vi "VI Linearisierung v2.vi"() -> ()   [LabVIEW 2020, in "Linearisierung v2.lvlib"] (continued)
              n1351 = Bundle("PDF Optionen (Ausgang)"=w2317, "postprocess"=w2327, w2306, "Pfad Auto Lin"=w2304, "File Name LIN"=w2293, "Pfad LIN"=w2292, "LIN Filename override"=w2291) -> (w2337:T200)  [unwired: 1 in]
              n1352 = Increment(x=w2300) -> (x+1=w2347:i32)
              n1353 = call "Auto Filenames.vi"("Fehler (Eingang)"=w2356, "Flags Cluster"=w2337, "Zeitstempel"=w2338, "SpanInletClusterArray in"=w2333) -> ("Fehler (Ausgang)"=w2336:errorcluster, "LogInfo-Cluster"=w2351:T196, "Pfad LIN Cluster"=w2303:cluster{"Pfad LIN SPAN":T9, "Pfad LIN":path}, "SpanInletClusterArray out"=w2335:T19[], "Span_Name"=w2343:string, "File Names"=w2340:T197)  [unwired: 2 out]
              n1354 = call "get Polynom and EPA Auswahl from SPAN and Comp Index.vi"("Component Index"=w2300, "SPAN Idx"=w2301) -> ("Index Cluster"=w2297:T189, "EPA Optionsfeld out"=w2298:T2, "Polynom-Ordnung out"=w2299:T55)  [unwired: 7 in]
              n1355 = call "Set SPAN Component.vi"("Protocol_only"=TRUE, "Gasnummer"=w2347, "Autolin Hovacal (alt)"=w2330, "Daten Hovacal (alt)"=w2329) -> ("error out"=w2355:errorcluster, "Gaskomponente"=w2314:T7, "LogInfo-Einstellung-Cluster"=w2350:T190, "Komponente"=w2348:string, "Einheit in String"=w2339:string)  [unwired: 3 in]
              n1356 = Unbundle(w2303) -> ("Pfad LIN SPAN"=w2296:T9, "Pfad LIN"=w2302:path)
              n1357 = Bundle("Komponente"=w2348, w2347, "Einheit in String"=w2339) -> (w2316:T191)  [unwired: 1 in]
              n1358 = call "Set SPAN Component Tables.vi"("EPA Optionsfeld"=w2298, "Polynom-Ordnung"=w2299, "error in (no error)"=w2355, "Gaskomponente"=w2314, "postprocess"=w2327, "Tabellenref."=w2328) -> ("EPA Ausgangs-Cluster"=w2353:T193, "LIN Ausgangs-Cluster"=w2312:T194, "Daten Aufzeichnen Ausgangs-Cluster"=w2354:T195, "Aktiv EPA"=w2325:T57, "Aktiv LIN"=w2326:bool[])  [unwired: 1 out]
              n1359 = Unbundle By Name(w2340) -> ("LIN TXT Datei Name"=w2341:string)
              n1360 = call "get SPAN component params EPA LIN.vi"("Index in"=w2297, "LIN Ausgangs-Cluster"=w2312, "Gaskomponente"=w2314, "Component"=w2316) -> ("Component Cluster"=w2315:T199)  [unwired: 4 in, 3 out]
              n1361 = Unbundle By Name(w2354) -> ("Ausgabetabelle"=w2324:T53, "Eingabetabelle behandelt"=w2323:string[][])
              n1362 = Unbundle By Name(w2312) -> ("LIN Ausgabetabelle"=w2322:string[][], "XY-Graph"=w2321:cluster{dbl[], dbl[]}[], "Polynomkoeff."=w2313:T198)
              n1363 = Unbundle By Name(w2353) -> ("EPA Ausgabetabelle"=w2319:string[][], "XY-Graph"=w2320:cluster{dbl[], dbl[]}[], "LINVer Auswertung"=w2318:string[][])
              n1364 = call "Postprocess Wrapper next SPAN Comp.vi"("Fehler (Eingang, kein Fehler)"=w2336, "reprocessing"=w2327, "SpanInletClusterArray in"=w2335) -> ("Fehler (Ausgang)"=w2334:errorcluster, "active postprocessing SPAN Component"=w2332:i32, "active postprocessing SPAN"=w2331:i32, "SpanInletClusterArray out"=w2307:T19[], "last postprocessing SPAN"=w2294:bool)  [unwired: 4 in]
              n1365 = Not(x=w2308) -> (.not. x?=w2305:bool)
              n1366 = call "FGV SPAN Verriegelung.vi"("aktion"=Aktion_FGV_SPAN_Verriegelung."setcomp", "Component Cluster"=w2315) -> ()  [unwired: 7 in, 3 out]
              n1367 = call "get SPAN Table MG.vi"("automatisch in"=w2295, "active reprocessing SPAN"=w2301, "SpanInletClusterArray in"=w2307) -> ("SpanComponentInfos-Cluster"=w2310:T186)  [unwired: 2 in, 6 out]
              n1368 = case shown="True" w2346 {
                tunnel: w2296 -> [_ w2362]
                tunnel: w2351 -> [_ w2361]
                tunnel: w2350 -> [_ w2360]
                tunnel: w2345 -> [_ w2359]
                tunnel: w2344 -> [_ w2358]
                tunnel: [_ w2357] -> _
                frame False {
                }
                frame True {
                  # "Error Log"
                  n1369 = call "Log SPAN autorun Errors.vi"("Sprachliste"=w2358, "Component Infos"=w2359, "LogInfo-Einstellung-Cluster"=w2360, "LogInfo-Cluster"=w2361, "Pfad LIN"=w2362) -> ("error out"=w2357:errorcluster)  [unwired: 6 in]
                }
              }
              n1370 = Select(t=w2311, s=w2305, f=w2310) -> (s? t:f=w2309:T186)
            }
          }
          "XY-Graph LIN 2" <- w2193
          "XY-Graph EPA 2" <- w2191
          n1371 = Not(x=w2179) -> (.not. x?=w2173:bool)
          n1372 = local write "LIN Polynomkoeffizienten"(w2194) -> ()
          n1373 = And(x=w2173, y=w2174) -> (x .and. y?=w2175:bool)
          n1374 = local write "Pfad Auto Lin"(w2159) -> ()
          n1375 = local write "Aktiv LIN"(w2199) -> ()
          n1376 = local write "Aktiv"(w2198) -> ()
          n1377 = local write "Ausgabetabelle"(w2197) -> ()
          n1378 = local write "Eingabetabelle"(w2196) -> ()
          n1379 = local write "LIN Ausgabetabelle"(w2195) -> ()
          n1380 = local write "XY-Graph LIN"(w2193) -> ()
          n1381 = local write "EPA Ausgabetabelle"(w2192) -> ()
          n1382 = local write "XY-Graph EPA"(w2191) -> ()
          n1383 = local write "EPA Auswertung"(w2190) -> ()
          n1384 = control-ref of="XY-Graph LIN 2"() -> (w2216:refnum<vi>)
          n1385 = control-ref of="XY-Graph EPA 2"() -> (w2215:refnum<vi>)
          n1386 = Select(t=w2176, s=w2175, f=w2178) -> (s? t:f=w2177:bool)
          n1387 = And(x=w2204, y=w2176) -> (x .and. y?=w2205:bool)
          n1388 = Bundle("SpanComponentInfos-Cluster"=w2181, "Span_Name"=w2211) -> (w2210:T201)  [unwired: 1 in]
          n1389 = case shown="False" w2205 {
            tunnel: w2209 -> [_ w2229]
            tunnel: [_ w2227] -> w2207
            tunnel: w2164 -> [w2221 w2228]
            tunnel: [w2221 w2226] -> w2158
            tunnel: w2206 -> [_ w2222]
            frame False {
            }
            frame True {
              n1390 = call "LIN speichern.vi"("File Name LIN"=w2229, "Pfad LIN"=w2228) -> ("error out"=w2227:errorcluster, ".LIN Datei Pfad"=w2224:path, "Pfad LIN out"=w2226:T9)  [unwired: 7 in]
              n1391 = Bundle("active postprocessing SPAN"=w2222, ".LIN Datei Pfad"=w2224) -> (w2223:T202)  [unwired: 1 in]
              n1392 = call "FGV Post Processing.vi"("Aktion"=Aktion_FGV_Post_Processing."filenames", "filenemas Cluster"=w2223) -> ()  [unwired: 6 in, 4 out]
            }
          }
          n1393 = Bundle("XY-Graph LIN 2"=w2216, "XY-Graph EPA 2"=w2215, "ResultPictures"=w2171, w2161) -> (w2214:T203)  [unwired: 1 in]
          n1394 = And(x=w2176, y=w2177) -> (x .and. y?=w2189:bool)
          n1395 = Select(t=enum16{"LIN", "EPA", "LIN + EPA"}."LIN", s=w2155, f=enum16{"LIN", "EPA", "LIN + EPA"}."LIN + EPA" ("LIN/EPA")) -> (s? t:f=w2156:enum16{"LIN", "EPA", "LIN + EPA"})
          n1396 = Select(t=w2156, s=w2163, f=enum16{"LIN", "EPA", "LIN + EPA"}."LIN" ("LIN/EPA")) -> (s? t:f=w2170:enum16{"LIN", "EPA", "LIN + EPA"})
          n1397 = Select(t=enum16{"LIN", "EPA", "LIN + EPA"}."EPA", s=w2160, f=w2170) -> (s? t:f=w2168:enum16{"LIN", "EPA", "LIN + EPA"})
          n1398 = call "PDF Protokolle gemeinsam.vi"("start"=w2189, "LIN/EPA"=w2168, "Pfad LIN"=w2158, "File Names"=w2208, "Graphs"=w2214, "Fehler (Eingang, kein Fehler)"=w2207, "SpanComponentInfos-Cluster"=w2210, "PDF Optionen"=w2183, "Polynom-Ordnung"=w2188) -> ("Fehler (Ausgang)"=w2166:errorcluster, "EPA Context (Ausgang)"=w2212:refnum<class "Context.lvclass">, "Context (Ausgang)"=w2213:refnum<class "Context.lvclass">)
          n1399 = call "FGV SPAN Verriegelung.vi"("aktion"=Aktion_FGV_SPAN_Verriegelung."Reset Save EPA redirect", "error in (no error)"=w2166) -> ("error out"=w2165:errorcluster)  [unwired: 7 in, 2 out]
        }
        n1400 = Not(x=w2038) -> (.not. x?=w2036:bool)
        n1401 = Not(x=w2037) -> (.not. x?=w2035:bool)
        n1402 = And(x=w2036, y=w2035) -> (x .and. y?=w2034:bool)
        n1403 = case shown="True" w2068 {
          tunnel: w2079 -> [w2379 _]
          tunnel: w2057 -> [_ w2399]
          tunnel: w2078 -> [w2374 w2397]
          tunnel: w2076 -> [w2364 w2396]
          tunnel: w2075 -> [w2363 w2395]
          tunnel: w2074 -> [w2377 w2394]
          tunnel: w2039 -> [_ w2393]
          tunnel: [w2373 _] -> _
          tunnel: w2060 -> [w2372 w2392]
          tunnel: w2067 -> [w2369 _]
          tunnel: w2066 -> [_ w2391]
          tunnel: w2066 -> [_ w2390]
          tunnel: w2048 -> [_ w2389]
          tunnel: w2038 -> [w2367 _]
          tunnel: w2044 -> [w2368 _]
          tunnel: w2043 -> [_ w2388]
          tunnel: w2034 -> [_ w2387]
          frame False {
            # "manuell"
            n1404 = Not(x=w2367) -> (.not. x?=w2365:bool)
            n1405 = case shown="Kein Fehler" w2369 {
              tunnel: ["Daten gespeichert!" ("String") "Fehler beim schreiben der Daten" ("String")] -> w2378
              frame No Error {
              }
              frame Error {
              }
            }
            n1406 = call "FGV SPAN Verriegelung.vi"("aktion"=Aktion_FGV_SPAN_Verriegelung."unlock") -> ("error out"=w2370:errorcluster)  [unwired: 8 in, 2 out]
            n1407 = Select(t=w2364, s=w2365, f=w2363) -> (s? t:f=w2366:refnum<class "Context.lvclass">)
            n1408 = call "ClosePage.vi"("popup viewer"=w2372, "Fehler (Eingang, kein Fehler)"=w2377, "Context (Eingang)"=w2366) -> ("Fehler (Ausgang)"=w2373:errorcluster)  [unwired: 8 in]
            n1409 = property class="Bool."(reference=w2374, error in=w2370, "DisabledEnum"=T66."Disabled and Grayed Out" ("Deaktiviert")) -> (error out=w2376:errorcluster)  [unwired: 1 out]
            n1410 = disable-structure shown="Deaktiviert" {
              disable-tunnel: w2368 -> [w2382 _]
              disable-tunnel: w2367 -> [w2381 _]
              frame Disabled {
                n1411 = case shown="False" w2381 {
                  tunnel: w2382 -> [w2383 w2384]
                  frame False {
                    n1412 = local write "Pfad LIN"(w2383) -> ()
                  }
                  frame True {
                    n1413 = local write "EPA Pfad"(w2384) -> ()
                  }
                }
              }
              frame Enabled {
              }
            }
            n1414 = call <vilib>:"Clear Errors.vi"("error in (no error)"=w2376) -> ()  [unwired: 5 in, 2 out]
            n1415 = call "Texte in VIs uebersetzen.vi"("Sprachliste"=w2379, "String zum Übersetzen"=w2378) -> ("String zum Übersetzen"=w2380:string)  [unwired: 9 in, 4 out]
            n1416 = One Button Dialog(message=w2380) -> ()  [unwired: 1 in, 1 out]
          }
          frame True {
            # "automatisch"
            n1417 = case shown="False" w2391 {
              tunnel: [Aktion_FGV_Spans_abarbeiten."lesen" ("Aktion") Aktion_FGV_Spans_abarbeiten."next" ("Aktion")] -> w2402
              frame False {
              }
              frame True {
              }
            }
            n1418 = call "FGV Spans abarbeiten.vi"("Aktion"=w2402, "SpanInletClusterArray in"=w2399) -> ("Comp Idx out"=w2398:i32, "active SPAN Idx out"=w2400:i32)  [unwired: 4 in, 4 out]
            n1419 = Less Than 0?(x=w2400) -> (x < 0?=w2401:bool)
            n1420 = case shown="True" w2401 {
              tunnel: w2398 -> [_ _]
              tunnel: w2397 -> [_ w2435]
              tunnel: w2396 -> [w2411 w2429]
              tunnel: w2395 -> [w2410 w2428]
              tunnel: w2394 -> [w2409 w2430]
              tunnel: w2393 -> [w2408 w2424]
              tunnel: [w2406 w2426] -> _
              tunnel: [w2407 w2427] -> _
              tunnel: [_ w2434] -> _
              tunnel: w2392 -> [w2405 w2431]
              tunnel: w2390 -> [_ w2432]
              tunnel: w2389 -> [_ w2423]
              tunnel: w2388 -> [_ w2422]
              tunnel: w2387 -> [_ w2421]
              frame False {
                # "weiter"
                n1421 = case shown="True" w2408 {
                  tunnel: w2411 -> [_ w2420]
                  tunnel: w2410 -> [_ w2419]
                  tunnel: w2409 -> [w2414 w2418]
                  tunnel: [w2414 w2417] -> w2407
                  tunnel: [w2414 w2416] -> w2406
                  tunnel: w2405 -> [_ w2415]
                  frame False {
                  }
                  frame True {
                    n1422 = call "ClosePage.vi"("popup viewer"=w2415, "Fehler (Eingang, kein Fehler)"=w2418, "Context (Eingang)"=w2420) -> ("Fehler (Ausgang)"=w2417:errorcluster)  [unwired: 8 in]
                    n1423 = call "ClosePage.vi"("popup viewer"=w2415, "Fehler (Eingang, kein Fehler)"=w2418, "Context (Eingang)"=w2419) -> ("Fehler (Ausgang)"=w2416:errorcluster)  [unwired: 8 in]
                  }
                }
                n1424 = property on="STARTEN" class="Bool. (strikt)"("Val(Sgnl)"=T4 TRUE ("Wert (signalisierend)")) -> (error out=w2412:errorcluster)  [unwired: 2 in, 1 out]
                n1425 = call <vilib>:"Clear Errors.vi"("error in (no error)"=w2412) -> ()  [unwired: 5 in, 2 out]
              }
              frame True {
                # "fertig"
                n1426 = call "FGV Spans abarbeiten.vi"("Aktion"=Aktion_FGV_Spans_abarbeiten."idle") -> ("error out"=w2433:errorcluster)  [unwired: 5 in, 5 out]
                n1427 = Or(x=w2423, y=w2424) -> (x .or. y?=w2425:bool)
                n1428 = case shown="False" w2432 {
                  tunnel: [w2447 w2471] -> w2434
                  tunnel: w2433 -> [w2448 w2470]
                  tunnel: w2431 -> [w2445 w2468]
                  tunnel: w2430 -> [w2444 w2465]
                  tunnel: w2429 -> [w2446 w2467]
                  tunnel: w2428 -> [w2443 w2466]
                  tunnel: [w2442 w2464] -> w2427
                  tunnel: [w2441 w2463] -> w2426
                  tunnel: w2425 -> [w2440 _]
                  tunnel: w2422 -> [_ w2462]
                  tunnel: w2421 -> [w2439 _]
                  frame False {
                    # "reprocessing next \noder fertig"
                    n1429 = case shown="False" w2439 {
                      tunnel: w2448 -> [w2450 w2453]
                      tunnel: [w2449 w2452] -> w2447
                      frame True {
                        n1430 = call "FGV Post Processing.vi"("Aktion"=Aktion_FGV_Post_Processing."next", "error in (no error)"=w2450) -> ("error out"=w2449:errorcluster)  [unwired: 6 in, 3 out]
                      }
                      frame False {
                        n1431 = call "FGV Post Processing.vi"("Aktion"=Aktion_FGV_Post_Processing."same", "error in (no error)"=w2453) -> ("error out"=w2452:errorcluster)  [unwired: 6 in, 3 out]
                      }
                    }
                    n1432 = case shown="True" w2440 {
                      tunnel: w2446 -> [_ w2461]
                      tunnel: w2445 -> [_ w2460]
                      tunnel: w2444 -> [w2455 w2459]
                      tunnel: w2443 -> [_ w2458]
                      tunnel: [w2455 w2457] -> w2442
                      tunnel: [w2455 w2456] -> w2441
                      frame False {
                      }
                      frame True {
                        n1433 = call "ClosePage.vi"("popup viewer"=w2460, "Fehler (Eingang, kein Fehler)"=w2459, "Context (Eingang)"=w2461) -> ("Fehler (Ausgang)"=w2457:errorcluster)  [unwired: 8 in]
                        n1434 = call "ClosePage.vi"("popup viewer"=w2460, "Fehler (Eingang, kein Fehler)"=w2459, "Context (Eingang)"=w2458) -> ("Fehler (Ausgang)"=w2456:errorcluster)  [unwired: 8 in]
                      }
                    }
                  }
                  frame True {
                    # "start\nreprocessing"
                    n1435 = local write "Pfad LIN"(w2462) -> ()
                    n1436 = local write "EPA Pfad"(w2462) -> ()
                    n1437 = call "FGV Post Processing.vi"("Aktion"=Aktion_FGV_Post_Processing."enable", "error in (no error)"=w2470) -> ("error out"=w2471:errorcluster)  [unwired: 6 in, 3 out]
                    n1438 = call "ClosePage.vi"("popup viewer"=w2468, "Fehler (Eingang, kein Fehler)"=w2465, "Context (Eingang)"=w2467) -> ("Fehler (Ausgang)"=w2464:errorcluster)  [unwired: 8 in]
                    n1439 = call "ClosePage.vi"("popup viewer"=w2468, "Fehler (Eingang, kein Fehler)"=w2465, "Context (Eingang)"=w2466) -> ("Fehler (Ausgang)"=w2463:errorcluster)  [unwired: 8 in]
                  }
                }
                n1440 = property class="Bool."(reference=w2435, "DisabledEnum"=T66."Disabled and Grayed Out" ("Deaktiviert")) -> (error out=w2437:errorcluster)  [unwired: 1 in, 1 out]
                n1441 = call <vilib>:"Clear Errors.vi"("error in (no error)"=w2437) -> ()  [unwired: 5 in, 2 out]
              }
            }
          }
        }
      }
      event Value Change {
        n1442 = event-data() -> ()  [unwired: 1 in, 1 out]
        n1443 = local read "Aktiv"() -> (w2482:T57)
        n1444 = call "EPA aktiv genug Punkte.vi"("Aktiv"=w2482) -> ()  [unwired: 9 in, 2 out]
        n1445 = case shown="True" TRUE {
          tunnel: w2478 -> [_ w2494]
          tunnel: w2477 -> [_ w2493]
          tunnel: w2476 -> [_ w2492]
          tunnel: w2475 -> [_ w2491]
          tunnel: w2474 -> [_ w2488]
          tunnel: w2473 -> [w2483 _]
          frame False {
            n1446 = call "Texte in VIs uebersetzen.vi"("Sprachliste"=w2483, "String zum Übersetzen"="EPA Test nicht gültig!\nMindestens 10 aktive Punkte nötig.\nPDF wurde nicht erzeugt" ("Nachricht")) -> ("String zum Übersetzen"=w2484:string)  [unwired: 9 in, 4 out]
            n1447 = One Button Dialog(message=w2484) -> ()  [unwired: 1 in, 1 out]
          }
          frame True {
            # "immer, auch wenn weniger als 10, wird im PDF eh angezeigt !"
            n1448 = call "Postprocessing aktiv.vi"() -> ("postprocess"=w2486:bool)  [unwired: 10 in, 1 out]
            n1449 = case shown="True" TRUE {
              tunnel: w2494 -> [_ _]
              tunnel: w2493 -> [_ _]
              tunnel: w2492 -> [_ _]
              tunnel: w2491 -> [_ _]
              tunnel: "EPA Pfad" -> [_ _]
              tunnel: "EPA Filename" -> [_ _]
              tunnel: w2488 -> [_ _]
              tunnel: w2486 -> [_ _]
              frame False {
                # "manuell - jetzt auch automatisiert !"
              }
              frame True {
                # "postprocessing ... wird im automatic abgehandelt (LIN Speichern)\n#EPA_Save_redirect\nNur mehr hier, da Postprocessing jetzt alles auf einmal speichert - EPA Speichern dann deaktiviert !\nUnd manuell geht auch mit Pfad in auto speichern ... der Dateiname wird soweiso nie genommen (aber dann angezeigt).\nmit #LinV2_auto_singleSave hier wieder aktiv ..."
                n1450 = call "FGV SPAN Verriegelung.vi"("aktion"=Aktion_FGV_SPAN_Verriegelung."Set Save EPA redirect") -> ("error out"=w2495:errorcluster)  [unwired: 8 in, 2 out]
                n1451 = property on="Speichern LIN" class="Bool. (strikt)"(error in=w2495, "Val(Sgnl)"=T4 TRUE ("Wert (signalisierend)")) -> (error out=w2498:errorcluster)  [unwired: 1 in, 1 out]
                n1452 = call <vilib>:"Clear Errors.vi"("error in (no error)"=w2498) -> ()  [unwired: 5 in, 2 out]
              }
            }
          }
        }
      }
      event Value Change {
        # "#LinV2_auto_singleSave"
        n1453 = event-data() -> ()  [unwired: 1 in, 6 out]
        n1454 = local read "Gasnummer LIN"() -> (w2501:T49)
        n1455 = Decrement(x=w2501) -> (x-1=w2502:T49)
        n1456 = call "MG FileName.vi"("Gasnummer:"=w2502) -> ("LIN TXT Datei Name"=w2503:string, "EPA TXT Datei Name"=w2504:string)  [unwired: 7 in, 2 out]
        n1457 = call "Preset Filenames.vi"("FileNameInput References"=w2499, "Filename Flag Cluster"=w2500, "LIN TXT Datei Name"=w2503, "EPA TXT Datei Name"=w2504) -> ()  [unwired: 8 in]
      }
      event Value Change {
        w2508 = T1 TRUE ("Wert")
        # "#LinV2_auto_singleSave"
        n1458 = event-data() -> ()  [unwired: 1 in, 6 out]
        n1459 = Unbundle(w2513) -> ("LIN Filename override"=w2512:refnum<vi>, "EPA Filename override"=w2511:refnum<vi>)
        n1460 = property class="Bool. (strikt)"(reference=w2512, "Value"=w2508) -> (error out=w2510:errorcluster)  [unwired: 1 in, 1 out]
        n1461 = property class="Bool. (strikt)"(reference=w2511, error in=w2510, "Value"=w2508) -> (error out=w2509:errorcluster)  [unwired: 1 out]
        n1462 = call <vilib>:"Clear Errors.vi"("error in (no error)"=w2509) -> ()  [unwired: 5 in, 2 out]
      }
      event Value Change {
        # "#Option10xSpanAuto ???"
        n1463 = event-data() -> ()  [unwired: 1 in, 1 out]
        n1464 = call "LinDaten speichern und laden.vi"("Aktion"=enum16{"speichern", "laden"}."speichern") -> ("error out"=w2527:errorcluster, "Setup Daten-Cluster"=w2520:T204)  [unwired: 4 in, 5 out]
        n1465 = Unbundle By Name(w2520) -> ("[Analyser]"=w2519:string)
        n1466 = call "LinDaten speichern und laden.vi"("Aktion"=enum16{"speichern", "laden"}."laden", "error in (no error)"=w2527, "test Polynom"=TRUE, "Analysator"=w2519) -> ("error out"=w2530:errorcluster, "LIN Protokoll Daten"=w2533:T119, "MessDaten Array"=w2532:string[][][], "Ident Cluster"=w2531:T205, "Setup Daten-Cluster"=w2525:T204, "Settings Cluster"=w2517:T206)  [unwired: 1 in, 1 out]
        n1467 = call "LIN Laden Errors.vi"("Fehler (Eingang, kein Fehler)"=w2530, "Ident Cluster"=w2531) -> ("error out"=w2529:errorcluster, "Error orccured"=w2526:bool, "LIN Loading Error Description Array"=w2524:T207, "Ident Cluster out"=w2523:T205)  [unwired: 5 in, 1 out]
        n1468 = case shown="True" w2526 {
          tunnel: w2520 -> [_ w2575]
          tunnel: w2525 -> [_ w2576]
          tunnel: w2524 -> [_ _]
          tunnel: w2523 -> [_ w2574]
          tunnel: [w2572 w2573] -> w2522
          frame False {
            w2572 = T4 TRUE  # CONTINUE
          }
          frame True {
            n1469 = call "show LIN Load Errors.vi"("loaded Setup Daten-Cluster"=w2576, "Ident Cluster"=w2574, "local Setup Daten-Cluster"=w2575) -> ("CONTINUE"=w2573:T4)  [unwired: 8 in]
          }
        }
        n1470 = case shown="True" w2522 {
          tunnel: w2533 -> [_ w2549]
          tunnel: w2532 -> [_ w2547]
          tunnel: w2529 -> [_ w2545]
          tunnel: w2517 -> [_ w2537]
          frame False {
          }
          frame True {
            # "Wie hier mit anderem Polynom verfahren ... und für MG alle Komp !?\nHier auswerten und Fehlermeldung ?!\nOder auch reinrechnen ?\n#Lin_Load_Polynom_Question"
            n1471 = call "Lin Daten aufarbeiten.vi"("Lin-Polynom"=w2549, "error in (no error)"=w2545, "Aktionen"=Aktion_Lin_Daten_aufarbeiten."Protkolldaten") -> ("error out"=w2548:errorcluster)  [unwired: 14 in, 10 out]
            n1472 = call "Lin Daten aufarbeiten.vi"("error in (no error)"=w2548, "TabellenArray"=w2547, "Aktionen"=Aktion_Lin_Daten_aufarbeiten."Nachbehandlung laden") -> ("error out"=w2546:errorcluster)  [unwired: 14 in, 10 out]
            n1473 = call "Komponentenausgabe.vi"("error in (no error)"=w2546) -> ("error out"=w2555:errorcluster, "Gaskomponente"=w2554:T7)  [unwired: 7 in, 2 out]
            n1474 = call "Lin Daten aufarbeiten.vi"("Index (Seite)"=w2554, "error in (no error)"=w2555, "Aktionen"=Aktion_Lin_Daten_aufarbeiten."lesen") -> ("TabellenArray"=w2553:string[][][], "Lin-Polynom"=w2538:T119, "error out"=w2539:errorcluster)  [unwired: 14 in, 8 out]
            n1475 = disable-structure shown="Deaktiviert" {
              disable-tunnel: w2553 -> [w2562 _]
              disable-tunnel: [w2558 w2568] -> w2543
              disable-tunnel: w2539 -> [w2557 w2569]
              disable-tunnel: w2538 -> [_ w2571]
              disable-tunnel: w2537 -> [_ w2570]
              frame Disabled {
                n1476 = for {
                  tunnel: w2562 -> [w2567] mode=indexing
                  tunnel: [w2563] -> w2560
                  stop <- w2564 stop-if-true
                  n1477 = call "Tabelle initialisieren.vi"("Neue Tabelle"=w2567) -> ("Tabelle"=w2566:string[][])  [unwired: 10 in]
                  n1478 = Array Size(array=w2566) -> (size(s)=w2565:i32[])
                  n1479 = Index Array(array=w2565) -> (element=w2563:i32)  [unwired: 1 in]
                  n1480 = Not Equal To 0?(x=w2563) -> (x != 0?=w2564:bool)
                }
                n1481 = call "LIN_EPA aktiv setzen.vi"("Anzahl aktiv"=w2560) -> ("Aktiv"=w2559:bool[][])  [unwired: 9 in, 1 out]
                n1482 = call "Lin Daten aufarbeiten.vi"("error in (no error)"=w2557, "LINArray"=w2559, "Aktionen"=Aktion_Lin_Daten_aufarbeiten."LIN/EPA aktiv laden", "EPA Array"=w2559) -> ("error out"=w2558:errorcluster)  [unwired: 13 in, 10 out]
              }
              frame Enabled {
                n1483 = call "LIN Laden nur Aktiv setzen.vi"("error in (no error)"=w2569, "LIN Protokoll Daten"=w2571, "Settings Cluster new"=w2570) -> ("error out"=w2568:errorcluster)  [unwired: 8 in]
              }
            }
            n1484 = control-ref of="passive Komponente:"() -> (w2544:refnum<vi>)
            n1485 = property class="Ring (strikt)"(reference=w2544, error in=w2543, "DisabledEnum"=T66."Enabled" ("Deaktiviert")) -> (error out=w2542:errorcluster)  [unwired: 1 out]
            n1486 = property on="Gasnummer Generieren" class="DigWert (strikt)"(error in=w2542, "Val(Sgnl)"=T49 1 ("Wert (signalisierend)")) -> (error out=w2540:errorcluster)  [unwired: 1 in, 1 out]
            n1487 = call <vilib>:"Clear Errors.vi"("error in (no error)"=w2540) -> ()  [unwired: 5 in, 2 out]
          }
        }
      }
      event Value Change {
        # "#LIN_only_save_Polynoms"
        n1488 = event-data() -> ()  [unwired: 1 in, 1 out]
        n1489 = call "Komponentenausgabe.vi"() -> ("Gaskomponente"=w2589:T7)  [unwired: 8 in, 3 out]
        n1490 = call "Lin Daten aufarbeiten.vi"("Index (Seite)"=w2589, "Aktiv"="Aktiv", "Aktionen"=Aktion_Lin_Daten_aufarbeiten."EPA aktiviert") -> ("Index (Seite) out"=w2582:i32, "error out"=w2590:errorcluster)  [unwired: 14 in, 9 out]
        n1491 = call "aktueller SPAN und Komponent Index.vi"() -> ("akt SPAN out"=w2577:i32)  [unwired: 7 in, 4 out]
        n1492 = call "LIN Polynom Ordnung oder Aktiv Changes für Postprocessing.vi"("Aktion"=Aktion_LIN_Polynom_Ordnung_ode_Aktiv_Changes_für_Postprocessing."schreiben", "active SPAN Idx"=w2577, "Changes"=TRUE) -> ()  [unwired: 5 in, 4 out]
        n1493 = call "Lin Daten aufarbeiten.vi"("Index (Seite)"=w2582, "error in (no error)"=w2590, "Aktionen"=Aktion_Lin_Daten_aufarbeiten."EPA auswerten") -> ("Index (Seite) out"=w2581:i32, "error out"=w2598:errorcluster)  [unwired: 14 in, 9 out]
        n1494 = call "Lin Daten aufarbeiten.vi"("Index (Seite)"=w2581, "error in (no error)"=w2598, "Aktionen"=Aktion_Lin_Daten_aufarbeiten."lesen") -> ("Eingabetabelle"=w2596:T54, "EPA Auswertung"=w2584:cluster{sgl[], sgl[], bool[]}, "error out"=w2597:errorcluster)  [unwired: 14 in, 8 out]
        n1495 = call "EPA_Tabelle zusammenbauen.vi"("error in (no error)"=w2597, "Eingabetabelle"=w2596) -> ("error out"=w2592:errorcluster, "XY-Graph"=w2593:cluster{dbl[], dbl[]}[], "EPA Ausgabetabelle"=w2595:string[][])  [unwired: 7 in]
        n1496 = control-ref of="EPA Auswertung"() -> (w2586:refnum<vi>)
        n1497 = call "FGV Auswertung sammeln.vi"("Aktion"=Aktion_FGV_Auswertung_sammeln."lesen", "error in (no error)"=w2592) -> ("LINVer Auswertung"=w2591:string[][])  [unwired: 7 in, 2 out]
        n1498 = Unbundle(w2584) -> (w2585:bool[])  [unwired: 2 out]
        n1499 = local write "EPA Ausgabetabelle"(w2595) -> ()
        n1500 = local write "EPA Auswertung"(w2591) -> ()
        n1501 = local write "XY-Graph EPA"(w2593) -> ()
        n1502 = call "Zellen einfaerben.vi"("Färben"=w2585, "Tabellenref."=w2586) -> ()  [unwired: 10 in]
      }
      event Value Change {
        # "#LIN_only_save_Polynoms"
        n1503 = event-data() -> ()  [unwired: 1 in, 1 out]
        n1504 = local read "Polynom-Ordnung"() -> (w2619:T55)
        n1505 = call "Komponentenausgabe.vi"() -> ("Gaskomponente"=w2614:T7)  [unwired: 8 in, 3 out]
        n1506 = call "aktueller SPAN und Komponent Index.vi"() -> ("akt SPAN out"=w2602:i32)  [unwired: 7 in, 4 out]
        n1507 = call "Lin Daten aufarbeiten.vi"("Index (Seite)"=w2614, "Aktiv"="Aktiv LIN", "Aktionen"=Aktion_Lin_Daten_aufarbeiten."LIN aktiviert") -> ("Index (Seite) out"=w2607:i32, "error out"=w2618:errorcluster)  [unwired: 14 in, 9 out]
        n1508 = call "LIN Polynom Ordnung oder Aktiv Changes für Postprocessing.vi"("Aktion"=Aktion_LIN_Polynom_Ordnung_ode_Aktiv_Changes_für_Postprocessing."schreiben", "active SPAN Idx"=w2602, "Changes"=TRUE) -> ()  [unwired: 5 in, 4 out]
        n1509 = call "Lin Daten aufarbeiten.vi"("Index (Seite)"=w2607, "error in (no error)"=w2618, "Polynom-Ordnung"=w2619, "Aktionen"=Aktion_Lin_Daten_aufarbeiten."Lin auswerten") -> ("Index (Seite) out"=w2606:i32, "error out"=w2617:errorcluster)  [unwired: 13 in, 9 out]
        n1510 = call "Lin Daten aufarbeiten.vi"("Index (Seite)"=w2606, "error in (no error)"=w2617, "Aktionen"=Aktion_Lin_Daten_aufarbeiten."lesen") -> ("Eingabetabelle"=w2615:T54, "Lin-Polynom"=w2612:T119)  [unwired: 14 in, 9 out]
        n1511 = Unbundle By Name(w2612) -> ("Polynomkoeff."=w2610:dbl[])
        n1512 = call "LinTabelle zusammenbauen.vi"("Eingabetabelle"=w2615) -> ("LIN Ausgabetabelle"=w2621:string[][])  [unwired: 7 in, 3 out]
        n1513 = Array To Cluster(array=w2610) -> (cluster=w2611:T185)
        n1514 = local write "LIN Polynomkoeffizienten"(w2611) -> ()
        n1515 = local write "LIN Ausgabetabelle"(w2621) -> ()
      }
      event "Boolsch für LinStart": Value Change {
        # "#Option10xSpanAuto"
        n1516 = event-data() -> ()  [unwired: 1 in, 1 out]
        n1517 = call "Test Status.vi"("Aktion"=Aktion_Test_Status."lesen") -> ("Tests sperren"=w2624:bool)  [unwired: 11 in, 3 out]
        n1518 = local read "Anforderung"() -> (w2626:T4)
        n1519 = control-ref of="Anforderung"() -> (w2631:refnum<vi>)
        n1520 = control-ref of="Status"() -> (w2630:refnum<vi>)
        n1521 = Not(x=w2624) -> (.not. x?=w2623:bool)
        n1522 = Or(x="Boolsch für LinStart", y="STARTEN") -> (x .or. y?=w2647:T4)
        n1523 = Compound Arithmetic op=AND ("Mehrfacharithmetik")(w2647, w2626, w2623) -> (w2641:T4)
        n1524 = property class="Bool."(reference=w2645, "DisabledEnum"=T66."Enabled" ("Deaktiviert")) -> (error out=w2644:errorcluster)  [unwired: 1 in, 1 out]
        n1525 = Bundle By Name(cluster=T152 {"Stufen Tabelle Array"=[], "auto Scan Points"=[], "Punkte umkehren"=[], "Parameterkontrolle Array"=[], "Eingabetabelle"=refnum, "Ausgabetabelle"=refnum, "Anforderung"=refnum, "Status Str Referenz"=refnum, "Prüfgasnamen Array"=[]} ("Referenzen Cluster"), "Stufen Tabelle Array"=w2638, "auto Scan Points"=w2637, "Punkte umkehren"=w2636, "Parameterkontrolle Array"=w2635, "Eingabetabelle"=w2634, "Ausgabetabelle"=w2632, "Anforderung"=w2631, "Status Str Referenz"=w2630, "Prüfgasnamen Array"=w2627) -> (w2633:T152)
        n1526 = case shown="False" w2642 {
          tunnel: [w2654 TRUE] -> w2646
          tunnel: w2641 -> [w2654 _]
          frame False {
          }
          frame True {
            # "#TestRun"
          }
        }
        n1527 = call "FGV Stoerungen sammeln und auswerten.vi"("Aktion"=Aktion_FGV_Stoerungen_sammeln_und_auswerten."lesen") -> ("Error"=w2650:bool)  [unwired: 12 in, 6 out]
        n1528 = call <vilib>:"Clear Errors.vi"("error in (no error)"=w2644) -> ()  [unwired: 5 in, 2 out]
        n1529 = case shown="True" w2646 {
          selector: w2646 -> [_ w2676]
          tunnel: w2652 -> [w2659 w2674]
          tunnel: w2650 -> [_ w2677]
          tunnel: w2636 -> [_ w2675]
          tunnel: [T4 FALSE ("STARTEN") _] -> w2640
          tunnel: w2633 -> [_ w2673]
          tunnel: w2630 -> [_ w2672]
          tunnel: w2626 -> [w2657 _]
          frame False {
            n1530 = case shown="True" w2657 {
              tunnel: w2659 -> [w2665 w2671]
              tunnel: [w2660 w2666] -> w2656
              frame False {
                # "keine Anforderung GD"
                n1531 = call "Texte in VIs uebersetzen.vi"("Sprachliste"=w2665, "String zum Übersetzen"="Keine Anforderung Gasteiler!" ("Status")) -> ("String zum Übersetzen"=w2661:string)  [unwired: 9 in, 4 out]
                n1532 = call "FGV Daten Abholung uebergeben.vi"("Zustand"=w2661, "Beendet"=FALSE, "Aktion"=Aktion_FGV_Daten_Abholung_uebergebenctl."schreiben") -> ("Zustand"=w2660:string)  [unwired: 8 in, 4 out]
              }
              frame True {
                # "anderer Test läuft gerade"
                n1533 = call "Texte in VIs uebersetzen.vi"("Sprachliste"=w2671, "String zum Übersetzen"="Anderer Test läuft gerade.\nBitte etwas Geduld." ("Status")) -> ("String zum Übersetzen"=w2667:string)  [unwired: 9 in, 4 out]
                n1534 = call "FGV Daten Abholung uebergeben.vi"("Zustand"=w2667, "Beendet"=FALSE, "Aktion"=Aktion_FGV_Daten_Abholung_uebergebenctl."schreiben") -> ("Zustand"=w2666:string)  [unwired: 8 in, 4 out]
              }
            }
            n1535 = local write "Status"(w2656) -> ()
          }
          frame True {
            n1536 = stacked-sequence {
              seq-local: [_ w2699 _ _ _ _] -> [_ _ w2792 w2818 w2827 _]
              tunnel: w2677 -> [w2682 _ _ _ _ _]
              tunnel: w2676 -> [w2681 _ _ _ _ _]
              tunnel: w2675 -> [_ w2710 _ _ _ _]
              tunnel: w2674 -> [_ w2700 _ _ _ _]
              tunnel: w2673 -> [_ w2697 _ _ _ _]
              tunnel: w2672 -> [_ w2706 _ _ _ _]
              frame #0 {
                w2683 = ""
                # "#Option10xSpanAuto"
                n1537 = disable-structure shown="Aktiviert" {
                  disable-tunnel: w2682 -> [w2687 _]
                  disable-tunnel: w2681 -> [w2686 _]
                  frame Disabled {
                    n1538 = And(x=w2687, y=w2686) -> (x .and. y?=w2691:bool)
                    n1539 = call "FGV Stoerungen sammeln und auswerten.vi"("Neustart"=w2691, "Aktion"=Aktion_FGV_Stoerungen_sammeln_und_auswerten."neustart") -> ("error out"=w2693:errorcluster)  [unwired: 11 in, 6 out]
                    n1540 = property on="FORTSETZEN" class="Bool."(error in=w2693, "Visible"=FALSE ("Sichtbar")) -> (error out=w2694:errorcluster)  [unwired: 1 in, 1 out]
                    n1541 = call <vilib>:"Clear Errors.vi"("error in (no error)"=w2694) -> ("error out"=w2692:errorcluster)  [unwired: 5 in, 1 out]
                    n1542 = call "FGV Stoerungen sammeln und auswerten.vi"("error in (no error)"=w2692, "Aktion"=Aktion_FGV_Stoerungen_sammeln_und_auswerten."reset error") -> ()  [unwired: 11 in, 7 out]
                  }
                  frame Enabled {
                    # "Würde Zustand in \"Lin Ver Daten zusammensammeln\" schon vorab parallel setzen ???\nSTART ist aber jetzt deaktiviert (könnte man bei GD Fehler zusammen mit Fortsetzen aktivieren ... aber sind die GD Fehler so stabil ?).\nFür AutoSPAN müsste der SPAN Next dann rückgängig gemacht werden ... wenn nur dre eine SPAN neugestartet werden soll,\naber es muss immer in diesem VI laufen, sonst fehlen alle Settings für das AutoSPAN - es darf nuiemals nicht in der Daten sammeln Schleife einfach weiter laufen ... \noder eben nur dort und hier darf dann aber nichts gemacht werden ... (HovaCAL fix Komponenten fehlen aber dann nach STBY ??? ) ???\nRIW 18.10.2023"
                  }
                }
                n1543 = local write "Status"(w2683) -> ()
                n1544 = call "FGV Daten Abholung uebergeben.vi"("Zustand"=w2683, "Anzeige aktualisieren"=FALSE, "Aktion"=Aktion_FGV_Daten_Abholung_uebergebenctl."schreiben") -> ("Zustand"=w2680:string, "error out"=w2679:errorcluster)  [unwired: 8 in, 3 out]
                n1545 = call "FGV GD Status Anzeige.vi"("Aktion"=Aktion_FGV_GD_Status_Anzeige."schreiben", "error in (no error)"=w2679, "Zustand in"=w2680) -> ()  [unwired: 7 in, 2 out]
              }
              frame #1 {
                # "#Option10xSpanAuto #AutorangeSpanfactorsOffsets #ALIN_Cancel_Save"
                n1546 = call "FGV GD Errors sammeln.vi"("Aktion"=Aktion_FGV_GD_Errors_sammeln."init") -> ("error out"=w2708:errorcluster)  [unwired: 8 in, 2 out]
                n1547 = local read "Gasteiler Span Eingänge"() -> (w2695:u16)
                n1548 = disable-structure shown="TestRun==TRUE" {
                  disable-tunnel: w2708 -> [w2784 w2791]
                  disable-tunnel: [w2783 w2791] -> w2707
                  frame condition #0 (active) {
                    # "#TestRun"
                    n1549 = disable-structure shown="Deaktiviert" {
                      disable-tunnel: w2784 -> [w2788 w2790]
                      disable-tunnel: [w2787 w2790] -> w2783
                      frame Disabled {
                        n1550 = call "FGV Stoerungen sammeln und auswerten.vi"("Errors"=T156 {"Störung Kommunikation"=FALSE, "Pressure carrier gas"=TRUE, "Pressure diluted gas"=FALSE, "Outlet Pressure"=TRUE, "SNOX before SAIR"=FALSE, "Störung Gasteiler"=FALSE}, "Aktion"=Aktion_FGV_Stoerungen_sammeln_und_auswerten."error") -> ()  [unwired: 11 in, 7 out]
                        n1551 = call "FGV GD Errors sammeln.vi"("Aktion"=Aktion_FGV_GD_Errors_sammeln."Test Data", "error in (no error)"=w2788) -> ("error out"=w2787:errorcluster)  [unwired: 7 in, 2 out]
                      }
                      frame Enabled {
                      }
                    }
                  }
                  frame condition #1 {
                  }
                }
                n1552 = call "FGV SpanEinstellungen.vi"("Aktion"=Aktion_FGV_SpanEinstellungen."lesen", "error in (no error)"=w2708) -> ("error out"=w2704:errorcluster, "automatisch out"=w2703:T20, "SpanInletClusterArray out"=w2705:T19[])  [unwired: 5 in, 2 out]
                n1553 = call "SPAN GD Test alle Formeln.vi"("GD Span Eingänge"=w2695, "Sprachliste"=w2700, "manueller SPAN Index in"=-1, "error in (no error)"=w2704, "automatisch in"=w2703, "Referenzen Cluster"=w2697, "SpanInletClusterArray in"=w2705) -> ("error out"=w2699:errorcluster, "automatisch out"=w2702:T20, "SpanInletClusterArray out"=w2701:T19[], "GD LNI Cluster"=w2698:T208)  [unwired: 1 in]
                n1554 = case shown="Kein Fehler" w2699 {
                  tunnel: w2710 -> [w2741 _]
                  tunnel: w2707 -> [w2740 _]
                  tunnel: w2706 -> [w2734 _]
                  tunnel: w2697 -> [w2732 _]
                  tunnel: w2702 -> [w2726 _]
                  tunnel: w2701 -> [w2725 _]
                  tunnel: w2700 -> [w2724 _]
                  tunnel: w2698 -> [w2723 _]
                  tunnel: w2695 -> [w2722 _]
                  frame No Error {
                    w2737 = FALSE  # manuelle Anforderung
                    w2730 = TRUE  # set Tables
                    # "#PDF_manu_MG"
                    n1555 = case shown="True" w2726 {
                      tunnel: w2725 -> [w2756 w2766]
                      tunnel: [w2758 w2763] -> w2746
                      tunnel: [w2757 w2759] -> w2738
                      tunnel: [w2752 w2765] -> w2743
                      tunnel: [w2751 w2764] -> w2736
                      tunnel: w2740 -> [_ _]
                      frame False {
                        w2751 = TRUE  # show Message
                        w2747 = 0 ("Index out")
                        n1556 = local read "Gasnummer Generieren"() -> (w2754:T49)
                        n1557 = call "is SPAN component active.vi"("Komponente"=w2754, "SPAN Idx"=w2747, "SpanInletClusterArray in"=w2756) -> ("aktiv?"=w2755:bool)  [unwired: 5 in, 3 out]
                        n1558 = call "get SPAN first active component.vi"("SPAN Idx"=w2747, "SpanInletClusterArray in"=w2756) -> ("error out"=w2748:errorcluster, "first aktive Komponente"=w2753:i32, "SPAN Idx out"=w2757:i32, "SpanInletClusterArray out"=w2758:T19[])  [unwired: 6 in]
                        n1559 = Decrement(x=w2754) -> (x-1=w2750:T49)
                        n1560 = call "LIN Polynom Ordnung oder Aktiv Changes für Postprocessing.vi"("Aktion"=Aktion_LIN_Polynom_Ordnung_ode_Aktiv_Changes_für_Postprocessing."init initial", "error in (no error)"=w2748, "active SPAN Idx"=w2747) -> ()  [unwired: 5 in, 4 out]
                        n1561 = Select(t=w2750, s=w2755, f=w2753) -> (s? t:f=w2752:i32)
                      }
                      frame True {
                        n1562 = call "FGV Spans abarbeiten.vi"("Aktion"=Aktion_FGV_Spans_abarbeiten."lesen") -> ("Comp Idx out"=w2767:i32, "active SPAN Idx out"=w2768:i32)  [unwired: 5 in, 4 out]
                        n1563 = Less Than 0?(x=w2768) -> (x < 0?=w2769:bool)
                        n1564 = case shown="True" w2769 {
                          tunnel: [w2773 w2775] -> w2759
                          tunnel: w2768 -> [w2773 _]
                          tunnel: w2766 -> [w2771 w2778]
                          tunnel: [w2772 w2781] -> w2765
                          tunnel: w2767 -> [w2772 _]
                          tunnel: [_ TRUE] -> w2764
                          tunnel: [w2771 w2778] -> w2763
                          frame False {
                          }
                          frame True {
                            n1565 = call "FGV Spans abarbeiten.vi"("Aktion"=Aktion_FGV_Spans_abarbeiten."start", "SpanInletClusterArray in"=w2778) -> ("Comp Idx out"=w2781:i32, "active SPAN Idx out"=w2775:i32)  [unwired: 4 in, 4 out]
                            n1566 = call "FGV Post Processing.vi"("Aktion"=Aktion_FGV_Post_Processing."init", "SpanInletClusterArray in"=w2778) -> ("error out"=w2776:errorcluster)  [unwired: 6 in, 3 out]
                            n1567 = local read "Pfad Auto Lin"() -> (w2774:T9)
                            n1568 = call "LIN Polynom Ordnung oder Aktiv Changes für Postprocessing.vi"("Aktion"=Aktion_LIN_Polynom_Ordnung_ode_Aktiv_Changes_für_Postprocessing."init initial", "error in (no error)"=w2776, "active SPAN Idx"=w2775) -> ()  [unwired: 5 in, 4 out]
                            n1569 = local write "Pfad LIN"(w2774) -> ()
                            n1570 = local write "EPA Pfad"(w2774) -> ()
                          }
                        }
                        n1571 = Bundle(cluster=T155 {"active postprocessing SPAN"=0, "active postprocessing SPAN Component"=0, "active postprocessing index"=0} ("active Index Cluster in"), "active postprocessing SPAN"=w2759) -> (w2760:T155)  [unwired: 2 in]
                        n1572 = call "FGV Post Processing.vi"("Aktion"=Aktion_FGV_Post_Processing."show", "active Index Cluster in"=w2760) -> ()  [unwired: 6 in, 4 out]
                      }
                    }
                    n1573 = call "FGV SPAN Verriegelung.vi"("active SPAN Index"=w2738, "aktion"=Aktion_FGV_SPAN_Verriegelung."lock") -> ("error out"=w2739:errorcluster)  [unwired: 7 in, 2 out]
                    n1574 = Bundle("manuelle Anforderung"=w2737, "show Message"=w2736, "set Tables"=w2730, "set Tables"=w2730) -> (w2735:T209)  [unwired: 1 in]
                    n1575 = call "Set actual ProtocolData from SPAN.vi"("Punkte umkehren Array"=w2741, "error in (no error)"=w2739, "Comp Idx"=w2743, "Index in"=w2738, "SpanInletClusterArray in"=w2746) -> ("error out"=w2744:errorcluster, "Index out"=w2731:i32, "SpanInletClusterArray out"=w2733:T19[])  [unwired: 3 in, 1 out]
                    n1576 = call "SPAN Stufen abfragen Gasteiler alle Komponenten.vi"("GD LNI Cluster"=w2723, "Sprachliste"=w2724, "Boolsche Flags Cluster"=w2735, "error in (no error)"=w2744, "Referenzen Cluster"=w2732, "SPAN Index in"=w2731, "SpanInletClusterArray in"=w2733) -> ("error out"=w2742:errorcluster, "Component Index out"=w2717:i32, "SPAN Index out"=w2712:i32, "SpanInletClusterArray out"=w2721:T19[], "Anzahl Stufen"=w2729:sgl)
                    n1577 = Bundle("SPAN Index out"=w2712, "Component Index out"=w2717) -> (w2716:T210)  [unwired: 1 in]
                    n1578 = call "SetHovaCAL_MFC_Concentration.vi"("error in (no error)"=w2742) -> ("error out"=w2728:errorcluster)  [unwired: 10 in]
                    n1579 = call "LIN Polynom Ordnung je Komponente für Protokoll.vi"("Aktion"=Aktion_LIN_Polynom_Ordnung_je_Komponente_für_Protokoll."init", "Index in"=w2716) -> ("error out"=w2720:errorcluster, "Index out"=w2715:T69)  [unwired: 3 in, 5 out]
                    n1580 = call "HovaCAL fix Sollwerte in Tabelle.vi"("error in (no error)"=w2728, "Anzahl Stufen"=w2729) -> ("error out"=w2727:errorcluster)  [unwired: 9 in]
                    n1581 = call "EPA Polynom Ordnung je Komponente für Protokoll.vi"("Aktion"=Aktion_EPA_Polynom_Ordnung_je_Komponente_für_Protokoll."init", "error in (no error)"=w2720, "Index in"=w2715) -> ("error out"=w2714:errorcluster)  [unwired: 4 in, 3 out]
                    n1582 = call "LIN Polynom Ordnung oder Aktiv Changes für Postprocessing.vi"("Aktion"=Aktion_LIN_Polynom_Ordnung_ode_Aktiv_Changes_für_Postprocessing."init", "error in (no error)"=w2714, "active SPAN Idx"=w2712) -> ()  [unwired: 5 in, 4 out]
                    n1583 = call "Aufschaltung CalGas Span.vi"("Status Str Referenz"=w2734, "Sprachliste"=w2724, "GD SPAN Eingänge"=w2722, "error in (no error)"=w2727, "Component Index"=w2717, "SPAN Index"=w2712, "SpanInletClusterArray"=w2721) -> ()  [unwired: 1 in, 4 out]
                  }
                  frame Error {
                  }
                }
              }
              frame #2 {
                # "#Neue_LIN"
                n1584 = case shown="Kein Fehler" w2792 {
                  frame No Error {
                    n1585 = call "Komponentenausgabe.vi"() -> ("error out"=w2793:errorcluster, "Gaskomponente"=w2795:T7)  [unwired: 8 in, 2 out]
                    n1586 = call "Lin Daten aufarbeiten.vi"("Index (Seite)"=w2795, "error in (no error)"=w2793, "Aktionen"=Aktion_Lin_Daten_aufarbeiten."lesen") -> ("Eingabetabelle"=w2796:T54, "error out"=w2798:errorcluster)  [unwired: 14 in, 9 out]
                    n1587 = call "AusgabeTabelle zusammenbauen.vi"("error in (no error)"=w2798, "Eingabetabelle"=w2796) -> ("error out"=w2810:errorcluster, "Eingabetabelle behandelt"=w2794:string[][], "Ausgabetabelle"=w2797:T53)  [unwired: 7 in]
                    n1588 = local write "Ausgabetabelle"(w2797) -> ()
                    n1589 = local write "Eingabetabelle"(w2794) -> ()
                    n1590 = call "Lin Daten aufarbeiten.vi"("error in (no error)"=w2810, "Aktionen"=Aktion_Lin_Daten_aufarbeiten."lesen") -> ("Lin-Polynom"=w2806:T119)  [unwired: 15 in, 10 out]
                    n1591 = Unbundle By Name(w2806) -> ("Lin Modus"=w2805:T10)
                    n1592 = case shown="1, Standard" w2805 {
                      tunnel: [Zustaende."Cal-Gas" ("Zustand") Zustaende."Messen" ("Zustand") Zustaende."Cal-Gas" ("Zustand") Zustaende."Cal-Gas" ("Zustand")] -> w2808
                      frame 1, Default {
                        # "Cal Gas to Samplepoint"
                      }
                      frame 2 {
                        # "Measure"
                      }
                      frame 3 {
                        # "Gasdivider"
                      }
                      frame 0 {
                        # "Cal Gas to PNS"
                      }
                    }
                    n1593 = call "FGV-Funktionstasten.vi"("Herkunft"="Linearisierung", "Zustand"=w2808, "Aktion"=Funktionstasten-Aktion."Zustand setzen") -> ("Fehler steht an"=w2800:bool)  [unwired: 5 in, 7 out]
                    n1594 = disable-structure shown="Deaktiviert" {
                      disable-tunnel: [w2812 _] -> w2801
                      disable-tunnel: w2800 -> [w2811 _]
                      frame Disabled {
                        # "UNKLAR !"
                        n1595 = call "warten.vi"("Datenfluss"=w2811, "Zu wartende ms"=u32 3000) -> ("error out"=w2812:errorcluster)  [unwired: 8 in, 1 out]
                      }
                      frame Enabled {
                      }
                    }
                    n1596 = call "FGV Gasteiler.vi"("error in (no error)"=w2801, "Aufzeichnung Start"=TRUE ("STARTEN"), "Aktionen"=Aktionen_FGV_Gasteiler_Daten."Aufzeichnung Start") -> ()  [unwired: 9 in, 8 out]
                  }
                  frame Error {
                  }
                }
              }
              frame #3 {
                # "warten bis GD Komm nicht mehr in Beenden\noder maximal 6 Zyklen der GD Komm"
                n1597 = case shown="Kein Fehler" w2818 {
                  frame No Error {
                    n1598 = while {
                      i -> [w2821]
                      stop <- w2822 stop-if-true
                      n1599 = Wait Until Next ms Multiple(millisecond multiple=u32 90 ("ms")) -> ()  [unwired: 1 out]
                      n1600 = call "FGV Daten Abholung uebergeben.vi"("Aktion"=Aktion_FGV_Daten_Abholung_uebergebenctl."lesen") -> ("Beendet"=w2825:bool)  [unwired: 10 in, 4 out]
                      n1601 = Not(x=w2825) -> (.not. x?=w2824:bool)
                      n1602 = Greater?(x=w2821, y=20) -> (0:w2820:bool)
                      n1603 = Or(x=w2824, y=w2820) -> (x .or. y?=w2822:bool)
                    }
                  }
                  frame Error {
                  }
                }
              }
              frame #4 {
